vi "To PDM task.vi"(10 "task":u64) -> (2 "PDM task":refnum<data-value>)   [LabVIEW 2022 SP3, in "DAAG task conversion.lvlib"]
uses:
  DAAG task conversion.lvlib
  <vilib>/PDM Acquisition Toolkit/host/Classes/Tasks/PDM Tasks/PDM Task.lvclass
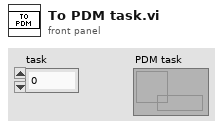
[diagram p1: front panel]
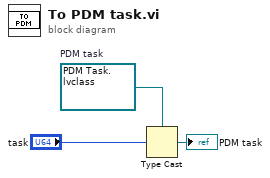
[diagram p0: block diagram]
diagram:
  w2 = refnum<data-value> refnum  # PDM task
  n1 = Type Cast(type=w2, x="task") -> (*(type *) &x=→"PDM task":refnum<data-value>)
